vi "read TBM configuration.vi"(8 "error in":errorcluster, 11 "Asynchronous Module Editor Node in":refnum<class "Asynchronous Module Editor Node.lvclass">) -> (0 "error out":errorcluster, 2 "configuration":refnum<class "TBM configuration.lvclass">, 3 "Asynchronous Module Editor Node out":refnum<class "Asynchronous Module Editor Node.lvclass">)   [LabVIEW 2013, in "Asynchronous Module Editor Node.lvclass"]
uses:
  Asynchronous Module Editor Node.lvclass
  <vilib>/NI/Tag Bus Module Framework/root configuration/TBM configuration.lvclass
  Asynchronous Module Editor Node.lvclass/Asynchronous Module Editor Node.ctl
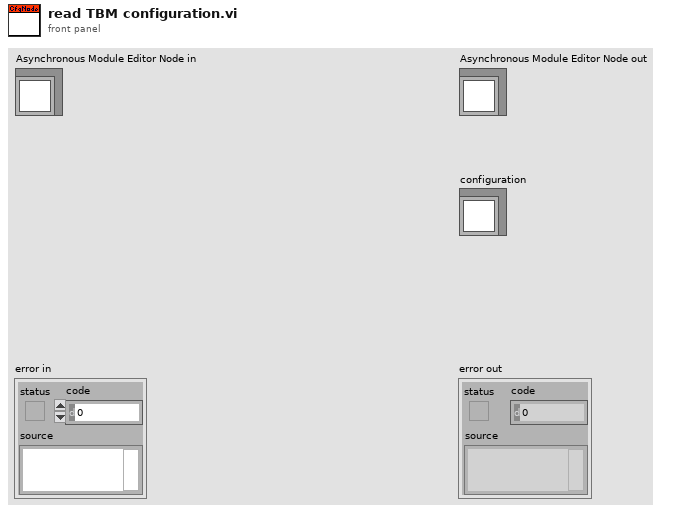
[diagram p1: front panel]
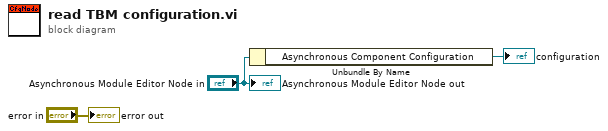
[diagram p0: block diagram]
diagram:
  n1 = Unbundle By Name("Asynchronous Module Editor Node in") -> ("Asynchronous Component Configuration"=→"configuration":refnum<class "asynchronous execution module configuration.lvclass">)
  "error out" <- "error in"
  "Asynchronous Module Editor Node out" <- "Asynchronous Module Editor Node in"
